vi "Configure Simple Frame.vi"(8 "error in":errorcluster, 10 "transfer ids":u16[](array[numeric]), 11 "module handle":u32) -> (0 "error out":errorcluster, 3 "module handle out":u32)   [LabVIEW 2020, in "AIM MIL-STD-1553 Hardware API.lvlib"]
uses:
  AIM MIL-STD-1553 Hardware API.lvlib
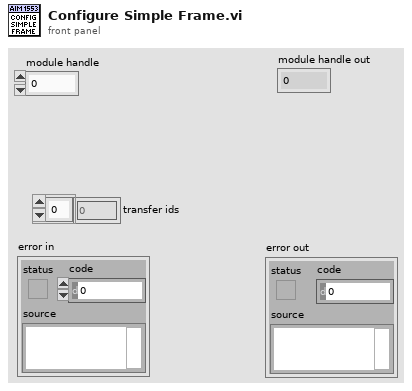
[diagram p1: front panel]
types:
  T1 = enum16{"n/a", "Normal transfer", "Skip (no op)", "Wait for time delay", "Strobe trigger"}
  T2 = cluster{"Instruction":enum16{"n/a", "Normal transfer", "Skip (no op)", "Wait for time delay", "Strobe trigger"}, "Numeric":u16}
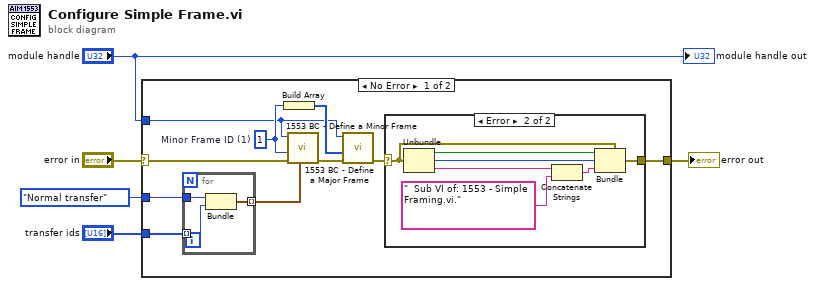
[diagram p0: block diagram]
diagram:
  n1 = case shown="No Error" "error in" {
    selector: "error in" -> [w14 w27]
    tunnel: [w7 w27] -> w5
    tunnel: "transfer ids" -> [w11 _]
    tunnel: T1."Normal transfer" ("Instruction") -> [w10 _]
    tunnel: "module handle" -> [w6 _]
    frame No Error {
      w13 = u8 1  # Minor Frame ID (1)
      n2 = for {
        tunnel: w11 -> [w17] mode=indexing
        tunnel: w10 -> [w18]
        tunnel: [w16] -> w9 mode=indexing
        n3 = Bundle("Instruction"=w18, "Numeric"=w17) -> (w16:T2)  [unwired: 1 in]
      }
      n4 = Build Array(w13) -> (w12:u8[])
      n5 = call <instrlib>:"1553 BC - Define a Minor Frame.vi"("Transfer List"=w9, "Error In (none)"=w14, "Minor Frame ID (1)"=w13, "Module Handle"=w6) -> ("Error Out"=w15:errorcluster)  [unwired: 6 in, 1 out]
      n6 = call <instrlib>:"1553 BC - Define a Major Frame.vi"("Error In (none)"=w15, "Frame List"=w12, "Module Handle"=w6) -> ("Error Out"=w8:errorcluster)  [unwired: 7 in, 1 out]
      n7 = case shown="Error" w8 {
        selector: w8 -> [w19 w26]
        tunnel: [w19 w23] -> w7
        frame No Error {
        }
        frame Error {
          n8 = Unbundle(w26) -> ("status"=w24:bool, "code"=w25:i32, "source"=w22:string)
          n9 = Concatenate Strings(w22, "  Sub VI of: 1553 - Simple Framing.vi.") -> (w21:string)
          n10 = Bundle(cluster=w26, "status"=w24, "code"=w25, "source"=w21) -> (w23:errorcluster)
        }
      }
    }
    frame Error {
    }
  }
  "error out" <- w5
  "module handle out" <- "module handle"
